vi "writeToXML.vi"(8 "error in (no error)":errorcluster, 10 "ClassLabel":string, 11 "CommandsForAllAxes in":refnum<class "CommandsForAllAxes.lvclass">) -> (0 "error out":errorcluster, 2 "XMLout":string, 3 "CommandsForAllAxes out":refnum<class "CommandsForAllAxes.lvclass">)   [LabVIEW 2014, in "TCSDataDefinitions.lvlib" / "TCSMountControlCommand.lvlib" / "CommandsForAllAxes.lvlib" / "CommandsForAllAxes.lvclass"]
uses:
  CommandsForAllAxes.lvclass
  TCSMCCCommand/TCSMCCCommand.lvclass
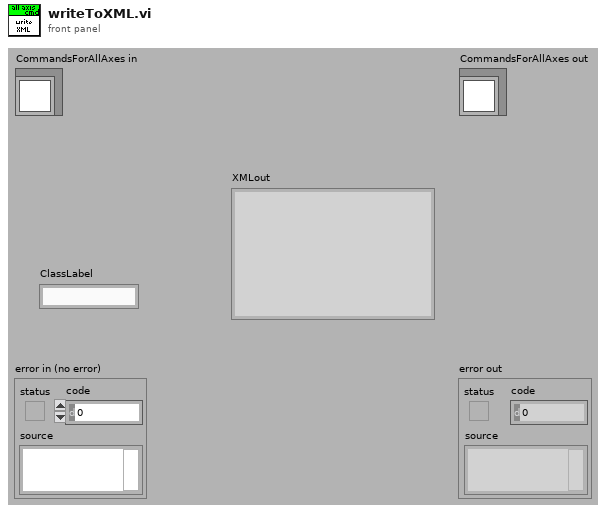
[diagram p1: front panel]
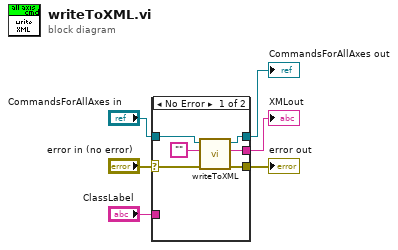
[diagram p0: block diagram]
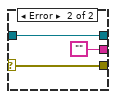
[diagram p2: hidden frame]
diagram:
  n1 = case shown="No Error" "error in (no error)" {
    selector: "error in (no error)" -> [w8 w15]
    tunnel: [w9 w15] -> w5
    tunnel: [w11 w14] -> w3
    tunnel: "CommandsForAllAxes in" -> [w12 w14]
    tunnel: [w10 ""] -> w2
    tunnel: "ClassLabel" -> [_ _]
    frame No Error {
      n2 = call-parent "writeToXML.vi"("error in (no error)"=w8, "ClassLabel"="", "TCSMCCCommand in"=w12) -> ("error out"=w9:errorcluster, "XMLout"=w10:string, "TCSMCCCommand out"=w11:refnum<class "CommandsForAllAxes.lvclass">)  [unwired: 6 in]
    }
    frame Error {
    }
  }
  "error out" <- w5
  "CommandsForAllAxes out" <- w3
  "XMLout" <- w2
